vi "fittingParams.vi"(6 "read/write":T3, 8 "error in (no error)":errorcluster, 9 "Coagulant":T4={"flocculator volume (L)"=100.0, "clarifier volume (L)"=0.0, "dose updates per HRT"=0, "target clarified turbidity (NTU)"=0.3, "Coagulant mode"=enum."manual", "Coag dose [mg/L]"=0.0, "pump mL/rev"=0.0} {"target clarified turbidity (NTU)" min=0.1 max=5.0 step=0.01; "dose updates per HRT" min=1 max=1000 step=1}, 10 "averaged data":T2) -> (0 "error out":errorcluster, 1 "Ccoag-DOM":dbl, 2 "Ku*":dbl, 3 "Fitting Params":cluster{dbl[], "Best Linear Fit":dbl[]}[](graph), 5 "coag model":T1)   [LabVIEW 2015]
uses:
  coag.ctl
  model type.ctl
  calcDoseorGetGraph.ctl
  data cluster.ctl
  Sensor buffer command.ctl
  coagbuffer.ctl
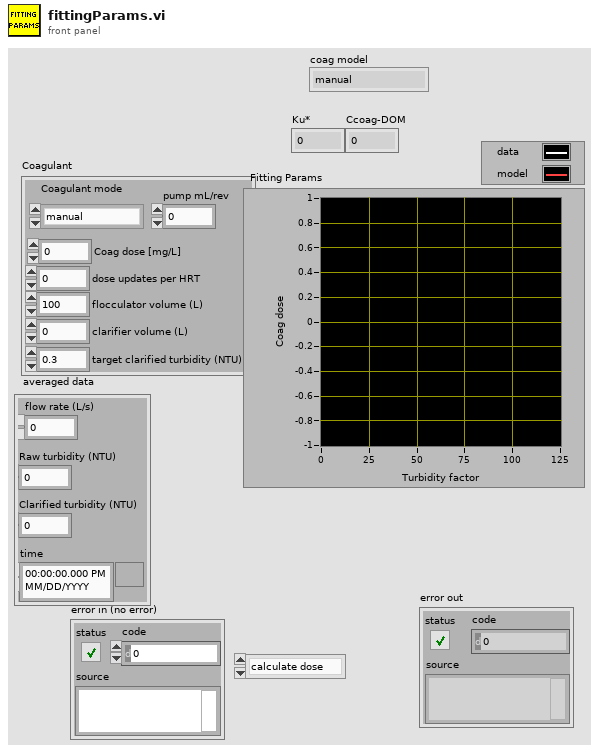
[diagram p1: front panel]
types:
  T1 = typedef "model type.ctl" = enum16{"manual", "simple corrector", "linear regression"}
  T2 = typedef "data cluster.ctl" = cluster{"Clarified turbidity (NTU)":dbl, "Raw turbidity (NTU)":dbl, "flow rate (L/s)":dbl, "time":timestamp}
  T3 = typedef "calcDoseorGetGraph.ctl" = enum16{"calculate dose", "read graph"}
  T4 = typedef "coag.ctl" = cluster{"flocculator volume (L)":dbl, "clarifier volume (L)":dbl, "dose updates per HRT":u32, "target clarified turbidity (NTU)":dbl, "Coagulant mode":T1, "Coag dose [mg/L]":dbl, "pump mL/rev":dbl}
  T5 = typedef "coagbuffer.ctl" = enum16{"set buffer size", "write", "refill buffer", "read recent", "read all", "clear", "overwrite"}
  T6 = typedef "Sensor buffer command.ctl" = enum16{"set buffer size", "write", "refill buffer", "read recent", "read all", "clear"}
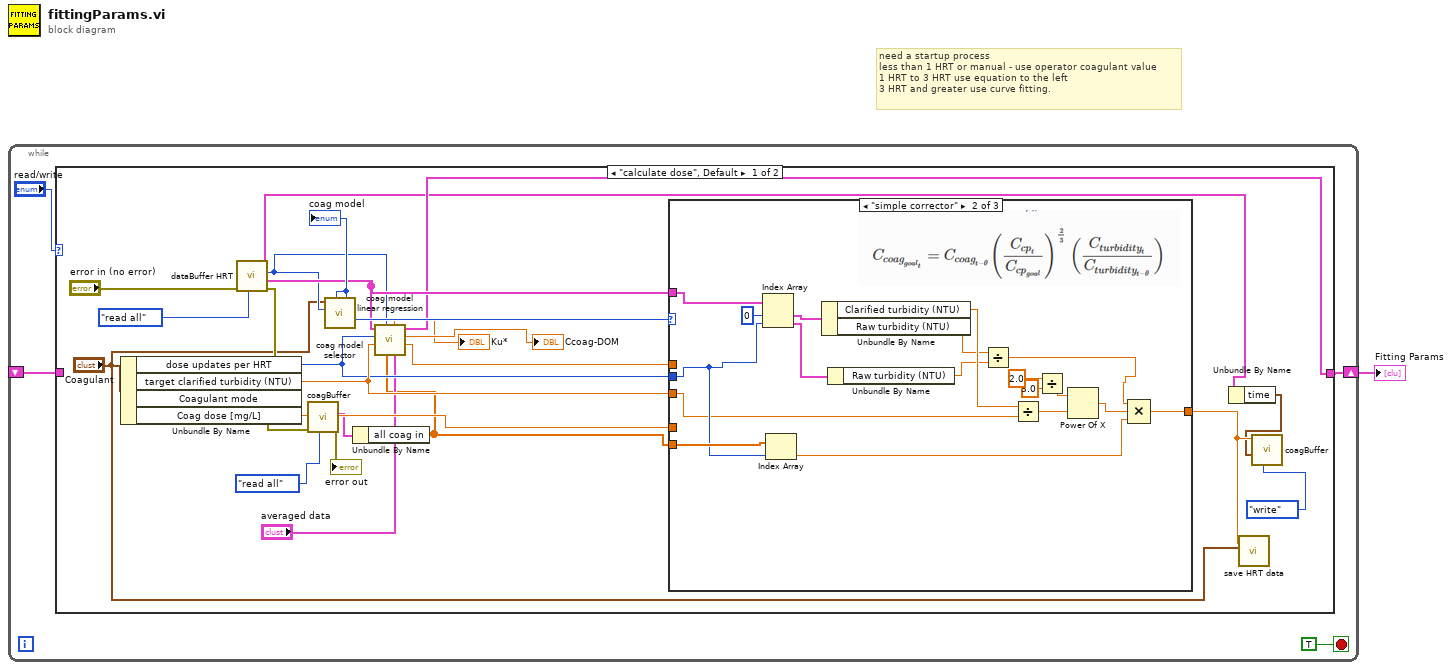
[diagram p0: block diagram]
diagram:
  # "need a startup process \nless than 1 HRT or manual - use operator coagulant value\n1 HRT to 3 HRT use equation to the left\n3 HRT and greater use curve fitting."
  n1 = while {
    shift-right: [w5] -> w1
    shift-left: _ -> [w4]
    stop <- TRUE stop-if-true
    n2 = case shown="\"calculate dose\", Default" "read/write" {
      tunnel: [w15 w49] -> w5
      tunnel: w4 -> [_ w49]
      frame "calculate dose", Default {
        n3 = Unbundle By Name("Coagulant") -> ("dose updates per HRT"=w18:u32, "target clarified turbidity (NTU)"=w19:dbl, "Coag dose [mg/L]"=w23:dbl)  [unwired: 1 out]
        n4 = call "dataBuffer HRT.vi"("command"=Sensor_buffer_command."read all", "error in (no error)"="error in (no error)") -> ("error out"=w26:errorcluster, "all data out"=w20:T2[], "scans"=w17:i32, "recent data"=w9:T2)  [unwired: 6 in]
        n5 = call "coagBuffer.vi"("command"=coagbuffer."read all", "error in (no error)"=w26) -> ("error out"=→"error out":errorcluster, "all data out"=w8:cluster{"time":timestamp[], "all coag in":dbl[]})  [unwired: 7 in, 1 out]
        n6 = call "coag model selector.vi"("scans"=w17, "Coagulant"="Coagulant") -> ("coag model"=w24:T1)  [unwired: 9 in]
        "coag model" <- w24
        n7 = Unbundle By Name(w8) -> ("all coag in"=w7:dbl[])
        n8 = call "coag model linear regression.vi"("averaged data"="averaged data", "all coag in"=w7, "scans"=w17, "target clarified turbidity (NTU)"=w19, "dose updates per HRT"=w18, "all data in"=w20) -> ("coag dose"=w16:dbl, "Ccoag-DOM"=→"Ccoag-DOM":dbl, "Graph"=w15:cluster{dbl[], "Best Linear Fit":dbl[]}[], "Ku*"=→"Ku*":dbl)  [unwired: 2 in]
        n9 = case shown="\"simple corrector\"" w24 {
          tunnel: w20 -> [_ w47 _]
          tunnel: w18 -> [_ w42 _]
          tunnel: w7 -> [_ w43 _]
          tunnel: w19 -> [_ w40 _]
          tunnel: [w29 w30 w48] -> w10
          tunnel: w23 -> [w29 _ _]
          tunnel: w16 -> [_ _ w48]
          frame "manual", Default {
          }
          frame "simple corrector" {
            n10 = Index Array(array=w47, index #1=0 ("index"), index #2=w42) -> (element #1=w45:T2, element #2=w44:T2)
            n11 = Index Array(array=w43, index=w42) -> (element=w31:dbl)
            n12 = Unbundle By Name(w45) -> ("Clarified turbidity (NTU)"=w41:dbl, "Raw turbidity (NTU)"=w35:dbl)
            n13 = Unbundle By Name(w44) -> ("Raw turbidity (NTU)"=w34:dbl)
            n14 = Divide(x=w35, y=w34) -> (x/y=w32:dbl)
            n15 = Divide(x=w41, y=w40) -> (x/y=w36:dbl)
            n16 = Divide(x=2.0, y=3.0) -> (x/y=w39:dbl)
            n17 = Power Of X(1:w36, 2:w39) -> (0:w33:dbl)
            n18 = Compound Arithmetic op=MULTIPLY(w32, w33, w31) -> (w30:dbl)
          }
          frame "linear regression" {
          }
        }
        n19 = Unbundle By Name(w9) -> ("time"=w6:timestamp)
        n20 = call "save HRT data.vi"("coagulant dose"=w10, "Coagulant"="Coagulant") -> ()  [unwired: 10 in]
        n21 = call "coagBuffer.vi"("command"=coagbuffer."write", "Time Stamp"=w6, "Coag dose"=w10) -> ()  [unwired: 6 in, 3 out]
      }
      frame "read graph" {
      }
    }
  }
  "Fitting Params" <- w1
